vi "RT to BC with Start Stop and Status.vi"(7 "base name for channel aliases":string, 8 "error in":errorcluster, 11 "Loopback in":refnum<class "Loopback.lvclass">) -> (0 "error out":errorcluster, 3 "Loopback out":refnum<class "Loopback.lvclass">)   [LabVIEW 2020, in "Loopback.lvclass"]
uses:
  Loopback.lvclass
  C:/Git/niveristand-custom-device-testing-tools/VeriStandTestCase/VeriStandTestCase.lvclass
  <vilib>/numeric/Random Number (Range) U64.vi
  cc108168-41e0-4b98-acb4-f1a10180548d.vi
  <vilib>/numeric/sub_Random U32.vi
  <vilib>/NI VeriStand/Execution/Workspace/NI VeriStand - Get Multiple Channel Values.vi
  <vilib>/NI VeriStand/Execution/Workspace/NI VeriStand - Set Single Channel Value.vi
  <vilib>/NI VeriStand/Execution/Workspace/NI VeriStand - Set Multiple Channel Values.vi
  niveristand-custom-device-testing-tools/VeriStandTestUtilities/VeriStandTestUtilities.lvlib
  <vilib>/NI VeriStand/Execution/Workspace/NI_VS Workspace ExecutionAPI.lvlib
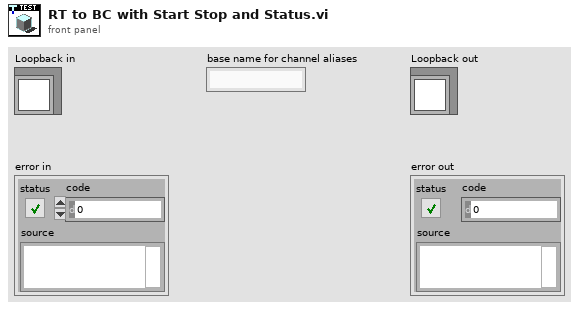
[diagram p1: front panel]
types:
  T1 = typedef "NI_VS Workspace ExecutionAPI.lvlib/WorkspaceAPI.ctl" = refnum<k24>
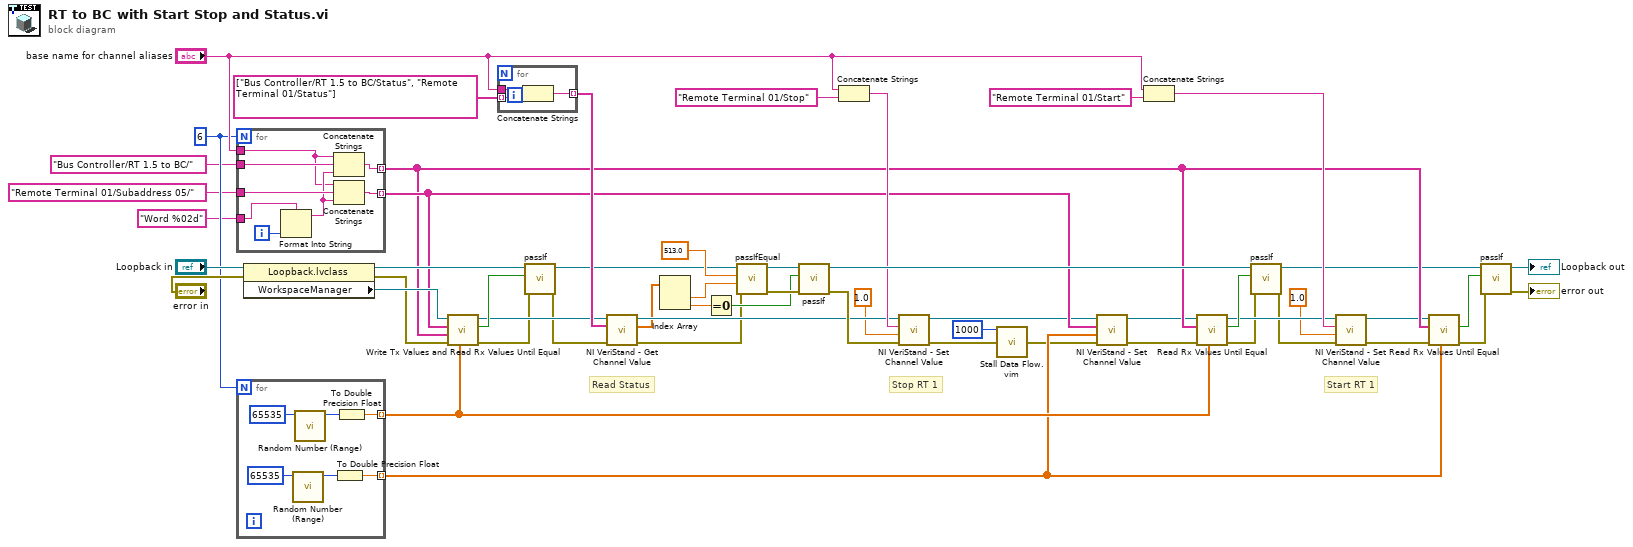
[diagram p0: block diagram]
diagram:
  w11 = 6
  # "Read Status"
  # "Start RT 1"
  # "Stop RT 1"
  n1 = for {
    N: w11 -> [_]
    tunnel: "Remote Terminal 01/Subaddress 05/" ("Channel") -> [w62]
    tunnel: [w63] -> w29 mode=indexing
    tunnel: "Bus Controller/RT 1.5 to BC/" ("Channel") -> [w61]
    tunnel: [w60] -> w28 mode=indexing
    tunnel: "Word %02d" -> [w57]
    tunnel: "base name for channel aliases" -> [w56]
    i -> [w59]
    n2 = Format Into String(format string=w57, w59) -> (resulting string=w58:string)  [unwired: 2 in, 1 out]
    n3 = Concatenate Strings(w56, w61, w58) -> (w60:string)
    n4 = Concatenate Strings(w56, w62, w58) -> (w63:string)
  }
  n5 = for {
    N: w11 -> [_]
    tunnel: [w67] -> w20 mode=indexing
    tunnel: [w64] -> w33 mode=indexing
    n6 = call-poly <vilib>:"Random Number (Range).vi"("upper bound (100)"=u64 65535) -> ("number"=w68:u64)  [unwired: 10 in]
    n7 = call-poly <vilib>:"Random Number (Range).vi"("upper bound (100)"=u64 65535) -> ("number"=w66:u64)  [unwired: 10 in]
    n8 = To Double Precision Float(number=w68) -> (double precision float=w67:dbl)
    n9 = To Double Precision Float(number=w66) -> (double precision float=w64:dbl)
  }
  n10 = property class="Loopback.lvclass"(reference="Loopback in", error in="error in") -> (reference out=w51:refnum<class "Loopback.lvclass">, error out=w52:errorcluster, "WorkspaceManager"=w53:T1)
  n11 = call "Write Tx Values and Read Rx Values Until Equal.vi"("Tx values"=w33, "error in"=w52, "Rx aliases"=w28, "Tx aliases"=w29, "workspace manager in"=w53) -> ("error out"=w30:errorcluster, "values equal"=w32:bool, "workspace manager out"=w31:T1)  [unwired: 4 in]
  n12 = for {
    tunnel: string[] ["Bus Controller/RT 1.5 to BC/Status", "Remote Terminal 01/Status"] -> [w72] mode=indexing
    tunnel: [w71] -> w37 mode=indexing
    tunnel: "base name for channel aliases" -> [w70]
    n13 = Concatenate Strings(w70, w72) -> (w71:string)
  }
  n14 = call-dynamic "passIf.vi"("error in (no error)"=w30, "pass"=w32, "TestCase in"=w51) -> ("error out"=w15:errorcluster, "TestCase out"=w16:refnum<class "Loopback.lvclass">)  [unwired: 7 in]
  n15 = call-poly <vilib>:"NI VeriStand - Get Channel Value.vi"("error in (no error)"=w15, "Channels"=w37, "WorkspaceManager in"=w31) -> ("error out"=w14:errorcluster, "Values"=w13:dbl[], "WorkspaceManager out"=w17:T1)  [unwired: 6 in]
  n16 = Index Array(array=w13) -> (element #1=w43:dbl, element #2=w45:dbl)  [unwired: 2 in]
  n17 = Equal To 0?(x=w45) -> (x = 0?=w46:bool)
  n18 = call-dynamic "passIfEqual.vi"("error in (no error)"=w14, "y"=w43, "x"=513.0 ("element"), "TestCase in"=w16) -> ("error out"=w47:errorcluster, "TestCase out"=w49:refnum<class "Loopback.lvclass">)  [unwired: 6 in]
  n19 = call-dynamic "passIf.vi"("error in (no error)"=w47, "pass"=w46, "TestCase in"=w49) -> ("error out"=w48:errorcluster, "TestCase out"=w50:refnum<class "Loopback.lvclass">)  [unwired: 7 in]
  n20 = Concatenate Strings("base name for channel aliases", "Remote Terminal 01/Stop" ("Channel")) -> (w39:string)
  n21 = call-poly <vilib>:"NI VeriStand - Set Channel Value.vi"("error in (no error)"=w48, "Value"=1.0, "Channel"=w39, "WorkspaceManager in"=w17) -> ("error out"=w9:errorcluster, "WorkspaceManager out"=w5:T1)  [unwired: 6 in]
  n22 = call "Stall Data Flow.vim"("value in"=w9, "milliseconds to wait"=u32 1000) -> ("value out"=w10:errorcluster)  [unwired: 1 out]
  n23 = call-poly <vilib>:"NI VeriStand - Set Channel Value.vi"("error in (no error)"=w10, "Values"=w20, "Channels"=w29, "WorkspaceManager in"=w5) -> ("error out"=w24:errorcluster, "WorkspaceManager out"=w23:T1)  [unwired: 6 in]
  n24 = Concatenate Strings("base name for channel aliases", "Remote Terminal 01/Start" ("Channel")) -> (w41:string)
  n25 = call "Read Rx Values Until Equal.vi"("expected values"=w33, "error in"=w24, "Rx aliases"=w28, "workspace manager in"=w23) -> ("error out"=w25:errorcluster, "values equal expected"=w27:bool, "workspace manager out"=w26:T1)  [unwired: 5 in]
  n26 = call-dynamic "passIf.vi"("error in (no error)"=w25, "pass"=w27, "TestCase in"=w50) -> ("error out"=w7:errorcluster, "TestCase out"=w12:refnum<class "Loopback.lvclass">)  [unwired: 7 in]
  n27 = call-poly <vilib>:"NI VeriStand - Set Channel Value.vi"("error in (no error)"=w7, "Value"=1.0, "Channel"=w41, "WorkspaceManager in"=w26) -> ("error out"=w19:errorcluster, "WorkspaceManager out"=w18:T1)  [unwired: 6 in]
  n28 = call "Read Rx Values Until Equal.vi"("expected values"=w20, "error in"=w19, "Rx aliases"=w28, "workspace manager in"=w18) -> ("error out"=w21:errorcluster, "values equal expected"=w22:bool)  [unwired: 5 in, 1 out]
  n29 = call-dynamic "passIf.vi"("error in (no error)"=w21, "pass"=w22, "TestCase in"=w12) -> ("error out"=→"error out":errorcluster, "TestCase out"=→"Loopback out":refnum<class "Loopback.lvclass">)  [unwired: 7 in]
